vi "2.1.-Lectura de Imagen - Extraer Capa RGB.vi"() -> ()   [LabVIEW 2020]
panel:
  out "2D Picture":picture
  in  "Path":path
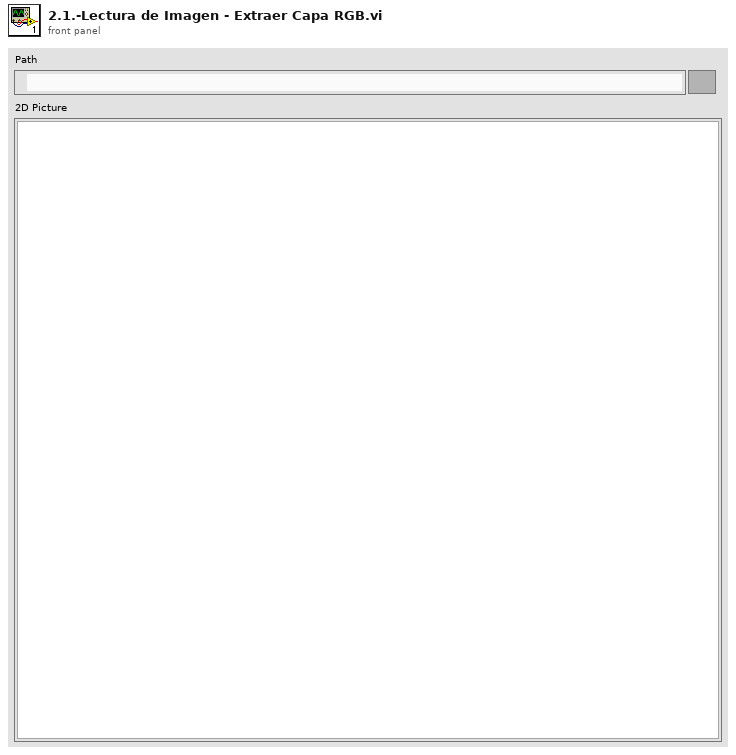
[diagram p1: front panel]
types:
  T1 = typedef "imagedata.ctl" = cluster{"image type":i32, "image depth":i32, "image":u8[], "mask":u8[], "colors":u32[], "Rectangle":cluster{"left":i16, "top":i16, "right":i16, "bottom":i16}}
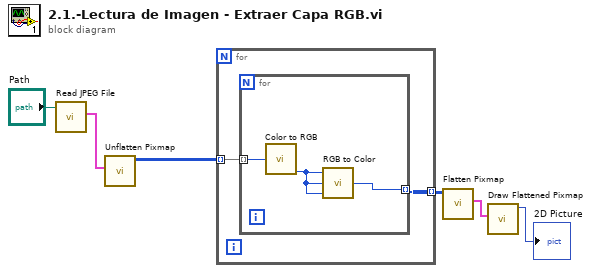
[diagram p0: block diagram]
diagram:
  n1 = call <vilib>:"Read JPEG File.vi"("path to JPEG file"="Path") -> ("image data"=w5:T1)  [unwired: 8 in, 2 out]
  n2 = call <vilib>:"Unflatten Pixmap.vi"("image data"=w5) -> ("24-bit pixmap"=w4:u32[][])  [unwired: 4 in, 6 out]
  n3 = for {
    tunnel: w4 -> [w8] mode=indexing
    tunnel: [w7] -> w3 mode=indexing
    n4 = for {
      tunnel: w8 -> [w11] mode=indexing
      tunnel: [w9] -> w7 mode=indexing
      n5 = call <vilib>:"Color to RGB.vi"("Color"=w11) -> ("B"=w10:u8)  [unwired: 3 out]
      n6 = call <vilib>:"RGB to Color.vi"("B"=w10, "G"=w10, "R"=w10) -> ("Color"=w9:u32)
    }
  }
  n7 = call <vilib>:"Flatten Pixmap.vi"("24-bit pixmap"=w3) -> ("image data"=w2:T1)  [unwired: 10 in]
  n8 = call <vilib>:"Draw Flattened Pixmap.vi"("image data"=w2) -> ("new picture"=→"2D Picture":picture)  [unwired: 8 in]
